vi "Create New IO Node.vi"(6 "Device Icon Name":string[](array[string]), 7 "Path to Analog Node Template":string="IONode\\Analog Input Node x.vi", 8 "error in":errorcluster, 9 "Device Alias":string, 10 "Values for Naming":T1={"Bus Number"=1, "Device Number"=1, "Channel Number"=1} {"Channel Number" min=1 step=1; "Device Number" min=1 step=1; "Bus Number" min=1 step=1}, 11 "Path to IO Node":path=path "D:/Documents/Projects/SPIAPI/IOEngineCode") -> (0 "error out":errorcluster, 2 "IO Node Name":string, 3 "Path to new IO Node":path)   [LabVIEW 2014, in "Initialization and IO Node Scripting.lvlib"]
uses:
  Initialization and IO Node Scripting.lvlib
  State Machine/Controls/Values for Naming.ctl
  Icon Editor/Icon Editor.llb/Icon Colors.ctl
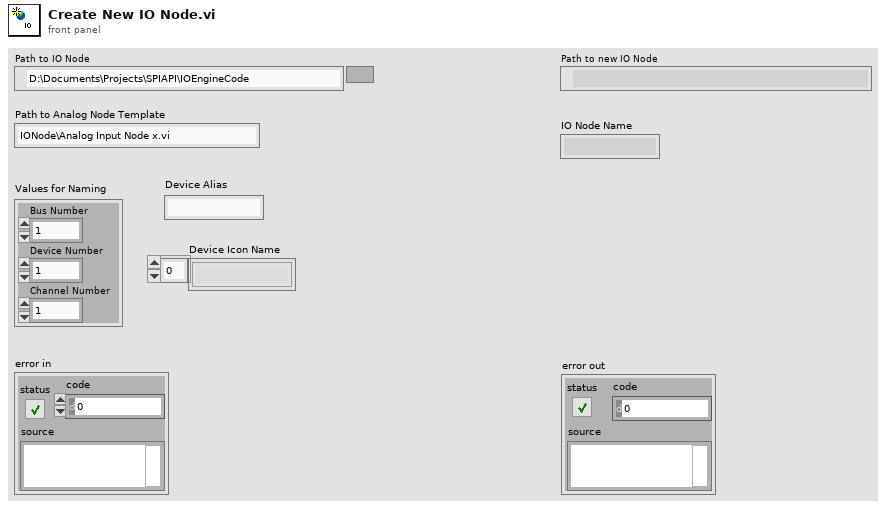
[diagram p1: front panel]
types:
  T1 = typedef "Initialization and IO Node Scripting.lvlib/Values for Naming.ctl" = cluster{"Bus Number":i32, "Device Number":i32, "Channel Number":i32}
  T2 = typedef "Initialization and IO Node Scripting.lvlib/Icon Colors.ctl" = cluster{"Text Color":u32, "Background Color":u32, "Border Color":u32}
  T3 = enum32{"invalid VI type", "Standard VI", "Control VI", "Global VI", "Polymorphic VI", "Configuration VI", "SubSystem", "Facade VI", "Method VI", "Statechart Diagram VI"}
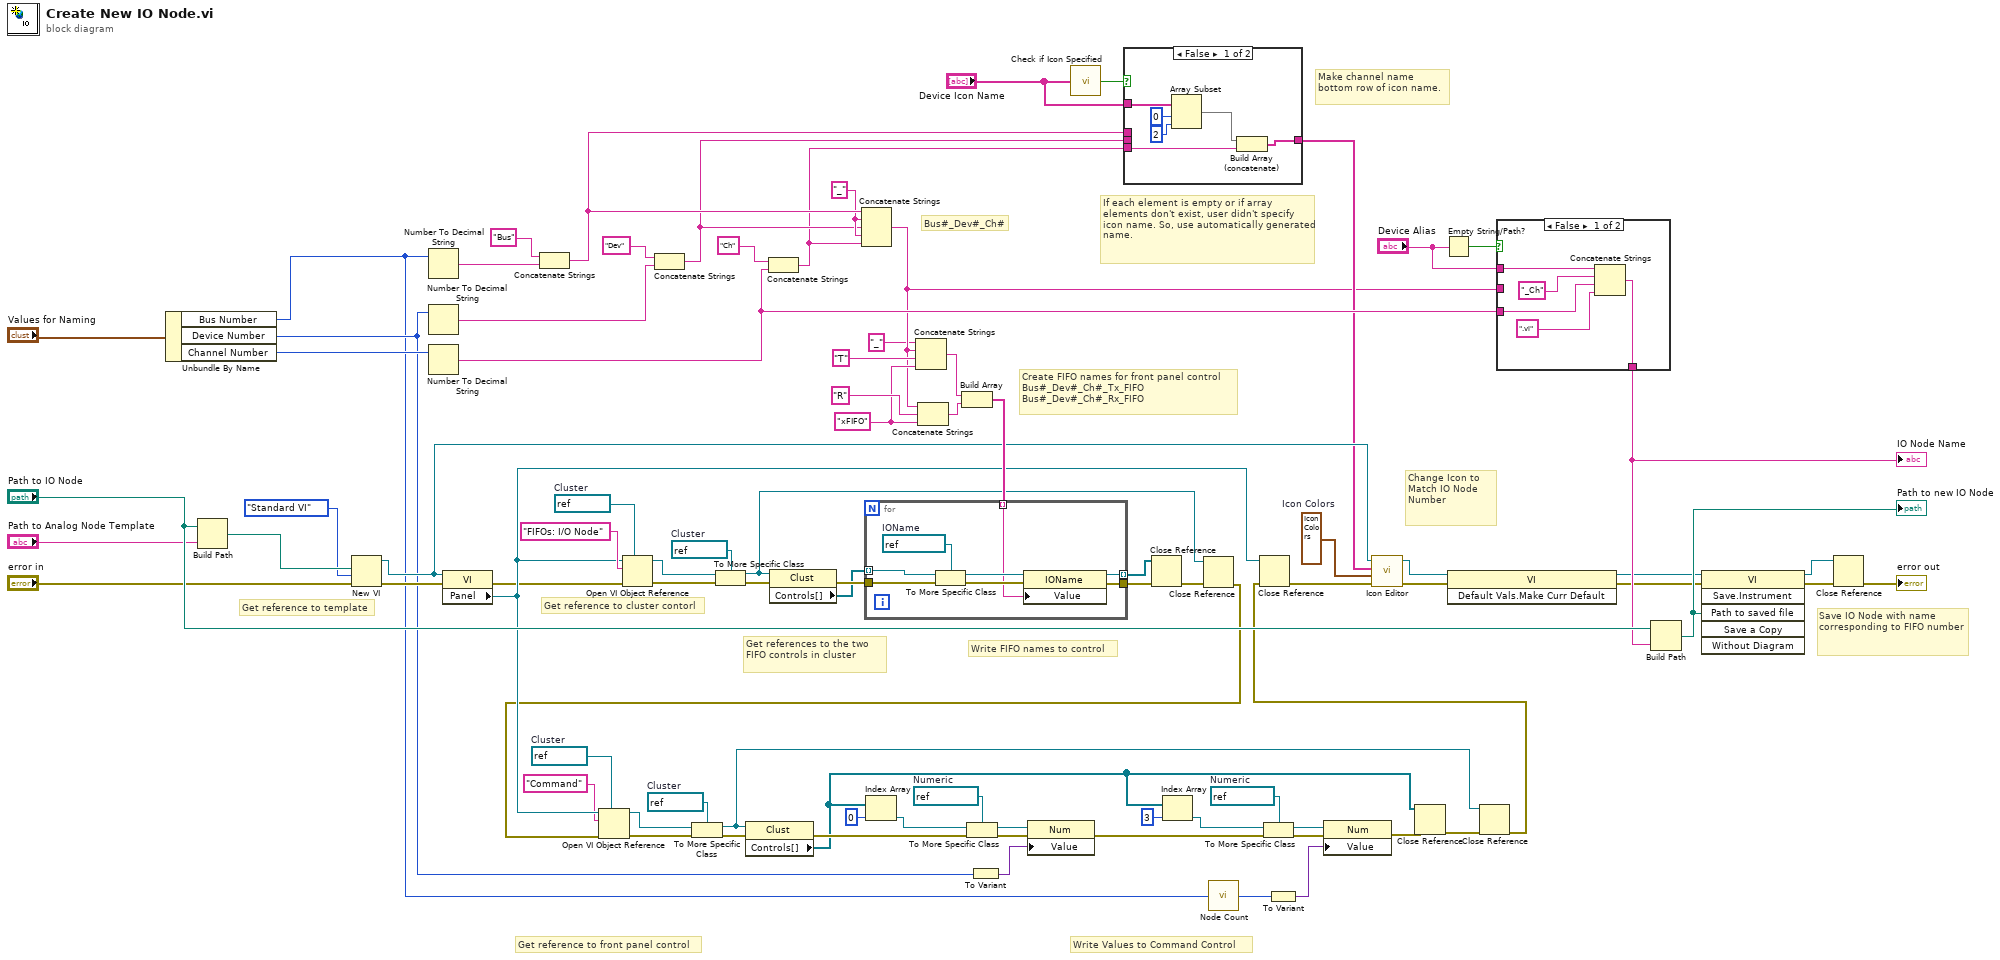
[diagram p0: block diagram]
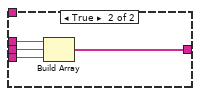
[diagram p3: hidden frame]
diagram:
  w5 = "_" ("string")
  w29 = refnum<vi> refnum  # Numeric
  w40 = refnum<vi> refnum  # Numeric
  w43 = refnum<vi> refnum  # Cluster
  w42 = refnum<vi> refnum  # Cluster
  w59 = T2 {"Text Color"=0, "Background Color"=16448250, "Border Color"=16746744}  # Icon Colors
  w65 = "xFIFO" ("string")
  w84 = refnum<vi> refnum  # Cluster
  w86 = refnum<vi> refnum  # Cluster
  # "Make channel name bottom row of icon name."
  # "If each element is empty or if array elements don't exist, user didn't specify icon name. So, use automatically generated name."
  # "Get reference to front panel control"
  # "Get references to the two FIFO controls in cluster"
  # "Write Values to Command Control"
  # "Bus#_Dev#_Ch#"
  # "Change Icon to Match IO Node Number"
  # "Get reference to template"
  # "Create FIFO names for front panel control\nBus#_Dev#_Ch#_Tx_FIFO\nBus#_Dev#_Ch#_Rx_FIFO"
  # "Save IO Node with name corresponding to FIFO number"
  # "Write FIFO names to control"
  # "Get reference to cluster contorl"
  n1 = Unbundle By Name("Values for Naming") -> ("Bus Number"=w25:i32, "Device Number"=w27:i32, "Channel Number"=w56:i32)
  n2 = Build Path(base path="Path to IO Node", name or relative path="Path to Analog Node Template") -> (appended path=w74:path)
  n3 = New VI(8:"error in", 9:T3."Standard VI" ("vi type (standard vi)"), 10:w74) -> (0:w85:errorcluster, 3:w60:refnum<vi>)  [unwired: 4 in]
  n4 = Number To Decimal String(number=w25) -> (decimal integer string=w50:string)  [unwired: 1 in]
  n5 = Number To Decimal String(number=w27) -> (decimal integer string=w49:string)  [unwired: 1 in]
  n6 = Number To Decimal String(number=w56) -> (decimal integer string=w18:string)  [unwired: 1 in]
  n7 = property class="VI"(reference=w60, error in=w85) -> (error out=w51:errorcluster, "Panel"=w52:refnum<vi>)  [unwired: 1 out]
  n8 = Concatenate Strings("Bus" ("string"), w50) -> (w6:string)
  n9 = Open VI Object Reference(7:w86, 8:w51, 10:"FIFOs: I/O Node" ("name/order"), 11:w52) -> (0:w83:errorcluster, 3:w82:refnum<vi>)
  n10 = Concatenate Strings("Dev" ("string"), w49) -> (w4:string)
  n11 = To More Specific Class(target class=w84, reference=w82, error in=w83) -> (specific class reference=w12:refnum<vi>, error out=w13:errorcluster)
  n12 = Concatenate Strings("Ch" ("string"), w18) -> (w3:string)
  n13 = property class="Clust"(reference=w12, error in=w13) -> (error out=w77:errorcluster, "Controls[]"=w70:refnum<vi>[])  [unwired: 1 out]
  n14 = Concatenate Strings(w6, w5, w4, w5, w3) -> (w2:string)
  n15 = Concatenate Strings("_" ("string"), w2, "T" ("name or relative path"), w65) -> (w63:string)
  n16 = Concatenate Strings(w2, "R" ("name or relative path"), w65) -> (w62:string)
  n17 = Build Array(w63, w62) -> (w69:string[])
  n18 = for {
    tunnel: [w94] -> w79 mode=indexing
    tunnel: [w93] -> w78
    tunnel: w77 -> [w89]
    tunnel: w70 -> [w88] mode=indexing
    tunnel: w69 -> [w87] mode=indexing
    w90 = refnum<vi> refnum  # IOName
    n19 = To More Specific Class(target class=w90, reference=w88, error in=w89) -> (specific class reference=w91:refnum<vi>, error out=w92:errorcluster)
    n20 = property class="IOName"(reference=w91, error in=w92, "Value"=w87) -> (reference out=w94:refnum<vi>, error out=w93:errorcluster)
  }
  n21 = To Variant(anything=w27) -> (Variant=w35:variant)
  n22 = call "Check if Icon Specified.vi"("Device Icon Name"="Device Icon Name") -> ("No Icon Specified"=w11:bool)
  n23 = case shown="False" w11 {
    tunnel: w6 -> [_ w104]
    tunnel: w4 -> [_ w103]
    tunnel: w3 -> [w96 w102]
    tunnel: [w95 w101] -> w9
    tunnel: "Device Icon Name" -> [w100 _]
    frame False {
      n24 = Array Subset(array=w100, index=0, length=2) -> (w97:string[])
      n25 = Build Array (concatenate)(w97, w96) -> (w95:string[])
    }
    frame True {
      n26 = Build Array(w104, w103, w102) -> (w101:string[])
    }
  }
  n27 = Close Reference(reference=w79, error in (no error)=w78) -> (error out=w80:errorcluster)
  n28 = Close Reference(reference=w12, error in (no error)=w80) -> (error out=w21:errorcluster)
  n29 = Open VI Object Reference(7:w42, 8:w21, 10:"Command" ("name/order"), 11:w52) -> (0:w45:errorcluster, 3:w46:refnum<vi>)
  n30 = To More Specific Class(target class=w43, reference=w46, error in=w45) -> (specific class reference=w41:refnum<vi>, error out=w44:errorcluster)
  n31 = property class="Clust"(reference=w41, error in=w44) -> (error out=w48:errorcluster, "Controls[]"=w23:refnum<vi>[])  [unwired: 1 out]
  n32 = Index Array(array=w23, index=0) -> (element=w38:refnum<vi>)
  n33 = To More Specific Class(target class=w40, reference=w38, error in=w48) -> (specific class reference=w37:refnum<vi>, error out=w36:errorcluster)
  n34 = property class="Num"(reference=w37, error in=w36, "Value"=w35) -> (error out=w28:errorcluster)  [unwired: 1 out]
  n35 = Index Array(array=w23, index=3) -> (element=w31:refnum<vi>)
  n36 = call "Node Count.vi"("Bus Number in"=w25) -> ("Node Number"=w26:i32)
  n37 = To More Specific Class(target class=w29, reference=w31, error in=w28) -> (specific class reference=w32:refnum<vi>, error out=w33:errorcluster)
  n38 = To Variant(anything=w26) -> (Variant=w34:variant)
  n39 = property class="Num"(reference=w32, error in=w33, "Value"=w34) -> (error out=w22:errorcluster)  [unwired: 1 out]
  n40 = Close Reference(reference=w23, error in (no error)=w22) -> (error out=w24:errorcluster)
  n41 = Empty String/Path?(string/path="Device Alias") -> (empty?=w8:bool)
  n42 = Close Reference(reference=w41, error in (no error)=w24) -> (error out=w20:errorcluster)
  n43 = Close Reference(reference=w52, error in (no error)=w20) -> (error out=w61:errorcluster)
  n44 = call "Icon Editor.vi"("Error In"=w61, "Icon Colors"=w59, "Text Array"=w9, "Reference to VI"=w60) -> ("Error Out"=w17:errorcluster, "Reference to VI"=w16:refnum<vi>)  [unwired: 6 in]
  n45 = invoke class="VI" method="Default Vals.Make Curr Default"(reference=w16, error in=w17) -> (reference out=w14:refnum<vi>, error out=w15:errorcluster)  [unwired: 1 in, 1 out]
  n46 = case shown="False" w8 {
    tunnel: [w109 w110] -> w19
    tunnel: w18 -> [w106 _]
    tunnel: "Device Alias" -> [w105 _]
    tunnel: w2 -> [_ w110]
    frame False {
      n47 = Concatenate Strings(w105, "_Ch" ("string"), w106, ".vi" ("string")) -> (w109:string)
    }
    frame True {
    }
  }
  "IO Node Name" <- w19
  n48 = Build Path(base path="Path to IO Node", name or relative path=w19) -> (appended path=w73:path)
  "Path to new IO Node" <- w73
  n49 = invoke class="VI" method="Save.Instrument"(reference=w14, error in=w15, "Path to saved file"=w73) -> (reference out=w72:refnum<vi>, error out=w76:errorcluster)  [unwired: 3 in, 4 out]
  n50 = Close Reference(reference=w72, error in (no error)=w76) -> (error out=→"error out":errorcluster)
